vi "keccak.ip.fifo.control.export.wrapper.vi"() -> ()   [LabVIEW 2021]
uses:
  <vilib>/Platform/TimedLoop/XDataNode/timing_clust.ctl
  <vilib>/Platform/TimedLoop/XDataNode/nitl_modes.ctl
  <vilib>/Platform/TimedLoop/XDataNode/wakeup.ctl
  <vilib>/rvi/Emulation/niFpgaSctlEmulationGetInTimedLoop.vi
  <vilib>/rvi/Emulation/niFpgaEmulationReportErrorSimple.vi
  <vilib>/rvi/Emulation/niFpgaGetClockAttributes.vi
  <vilib>/rvi/Emulation/niFpgaCriticalErrorInLSC.vi
  <vilib>/rvi/interface/RandomDataEmulation/niFpgaRandomDataHandleErrors.vi
  <vilib>/platform/TimedLoop/XDataNode/XDataNode.xnode
  <vilib>/rvi/DataTransferAndStorage/Container/XNode/niFpgaContainer.xnode
  <vilib>/rvi/interface/RandomDataEmulation/nirviRandomDataFpgaReadWriteTemplate.vi
  <vilib>/Platform/TimedLoop/XDataNode/XDNodeRunTimeDep.lvlib
panel:
  in  "Reset":bool
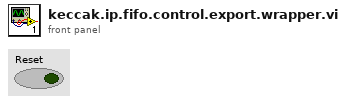
[diagram p1: front panel]
types:
  T1 = typedef "XDNodeRunTimeDep.lvlib/timing_clust.ctl" = cluster{"Expected End [f-1]":u64, "Actual End [f-1]":u64, "Finished Late? [f-1]":bool, "Expected End [i-1]":u64, "Actual End [i-1]":u64, "Finished Late? [i-1]":bool, "Expected Start [i]":u64, "Actual Start [i]":u64, "Expected Start [f]":u64, "Actual Start [f]":u64, "Source Name":string, "Structure Name":string, "Period":i64, "Deadline":i64, "Offset":i64, "Start":i64, "Priority":i32, "Timeout":i32, "Mode":T2, "Wakeup Reason":T3, "Error":errorcluster, "Source Type":string, "Secondary Source Type":string, "Global End Time":u64, "Global Start Time":u64, "Frame Duration":u64, "Iteration Duration":u64, "Assigned CPU":i32, "I/O Scan Engine Mode":u32}
  T2 = typedef "XDNodeRunTimeDep.lvlib/nitl_modes.ctl" = enum32{"No Change", "Process missed periods, maintain original phase", "Discard missed periods, maintain original phase", "Process missed periods, ignore original phase", "Discard missed periods, ignore original phase"}
  T3 = typedef "XDNodeRunTimeDep.lvlib/wakeup.ctl" = enum32{"Normal", "Aborted", "Asynchronous wakeup", "Timing source error", "Timed loop error", "Timeout"}
  T4 = cluster{"TS_RESULTS.Ready":bool, "TS_PARMS.Element":u64, "TS_PARMS.Valid":bool, "TS_DATA.Element":u64, "TS_DATA.Valid":bool}
  T5 = cluster{"TS_RESULTS.Element":u64, "TS_RESULTS.Valid":bool, "TS_PARMS.Ready":bool, "TS_DATA.Ready":bool}
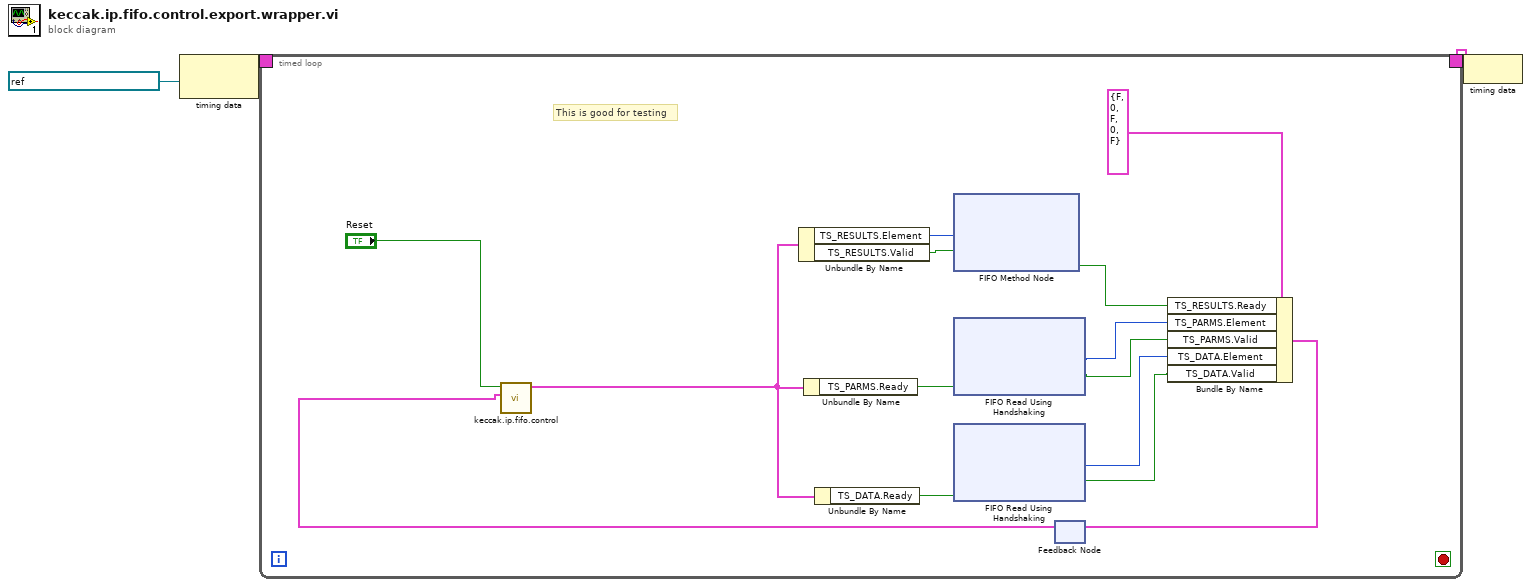
[diagram p0: block diagram]
diagram:
  n1 = node-c288(refnum<k21> "40 MHz Onboard Clock" ("Source Name")) -> (w3:T1)
  n2 = timed-loop {
    timing: w3 -> [_]
    timing-out: [_] -> w2
    stop <- _ stop-if-true
    # "This is good for testing"
    n3 = feedback #1() -> (w6:T4)  [unwired: 1 in]
    n4 = call "keccak.ip.fifo.control.vi"("FIFO.inputs"=w6, "Reset"="Reset") -> ("FIFO.outputs"=w5:T5)  [unwired: 9 in]
    n5 = Unbundle By Name(w5) -> ("TS_RESULTS.Element"=w17:u64, "TS_RESULTS.Valid"=w16:bool)
    n6 = Unbundle By Name(w5) -> ("TS_PARMS.Ready"=w15:bool)
    n7 = Unbundle By Name(w5) -> ("TS_DATA.Ready"=w14:bool)
    n8 = xnode ("FIFO Method Node")("Element"=w17, "Input Valid"=w16) -> ("Ready for Input"=w12:bool)  [unwired: 1 in, 1 out]
    n9 = xnode ("FIFO Read Using Handshaking")("Ready for Output"=w15) -> ("Element"=w11:u64, "Output Valid"=w10:bool)  [unwired: 1 in, 1 out]
    n10 = xnode ("FIFO Read Using Handshaking")("Ready for Output"=w14) -> ("Element"=w9:u64, "Output Valid"=w8:bool)  [unwired: 1 in, 1 out]
    n11 = Bundle By Name(cluster=T4 {"TS_RESULTS.Ready"=FALSE, "TS_PARMS.Element"=0, "TS_PARMS.Valid"=FALSE, "TS_DATA.Element"=0, "TS_DATA.Valid"=FALSE} ("FIFO.inputs"), "TS_RESULTS.Ready"=w12, "TS_PARMS.Element"=w11, "TS_PARMS.Valid"=w10, "TS_DATA.Element"=w9, "TS_DATA.Valid"=w8) -> (w7:T4)
    n12 = feedback-in #1(w7) -> ()
  }
  n13 = node-c288(w2) -> ()
